vi "Nonlinear Lev-Mar Fit.vi"(5 "derivative":T2(ring), 6 "Standard Deviation":dbl[](array[numeric]) format="%0.2f", 7 "max iteration":i32=200, 8 "Initial Guess Coefficients":dbl[](array[numeric]) format="%0.2f", 9 "Y":dbl[](array[numeric]) format="%0.2f", 10 "X":dbl[](array[numeric]) format="%0.2f") -> (0 "error":i32, 1 "mse":dbl format="%0.4e", 2 "Best Fit":dbl[](array[numeric]) format="%0.2f", 3 "Best Fit Coefficients":dbl[](array[numeric]) format="%0.2f", 4 "Covariance":T1)   [LabVIEW 2014, in "NI_AALPro.lvlib"]
doc: "LabVIEW no longer supports this VI. Use the Nonlinear Curve Fit VI instead.\n\nUses the Levenberg-Marquardt algorithm to determine the least squares set of coefficients that best fit the set of input data points (X,Y) as expressed by a nonlinear function y=f(x,a), where a is the set of coefficients.\n\nUnlike the Levenberg Marquardt VI, you cannot wire formula strings representing models directly to this VI. You have to specify the nonlinear functions within a subVI of this VI. If you can express the models as formula strings, use the Levenberg Marquardt VI. If the Levenberg Marquardt VI takes too long to run because you have a large number of points, or if you cannot express your models as formula strings, use the Nonlinear Lev-Mar Fit VI instead.\n\nThis VI assumes that you have prior knowledge of the nonlinear relationship between the x and y coordinates. That is, f = f(X, A), where the set of coefficients, A, is determined by the Levenberg-Marquardt algorithm.\n\nIf your values of x are too large, consider normalizing them before applying them to this VI.\n\nYou must specify the nonlinear function f = f(X, A) in the Formula Node on the block diagram of the Target Fnc & Deriv NonLin VI, which is a subVI of the Nonlinear Lev-Mar Fit VI. To access the Target Fnc & Deriv NonLin VI, select <b>View>>Browse Relationships>>This VI's SubVIs>>Target Fnc & Deriv NonLin.vi</b>.\n\nThis VI provides the following two methods to calculate the Jacobian (partial derivatives with respect to the coefficients) needed in the algorithm:\n<b>numerical calculation</b> uses a numerical approximation to compute the Jacobian.\n<b>formula calculation</b> uses a formula to compute the Jacobian. You need to specify the Jacobian function df/dA in the Formula Node on the block diagram of the Target Fnc & Deriv NonLin VI, as well as the nonlinear function f = f(X, A) This is a more efficient computation than the numerical calculation, because it does not require a numerical approximation to the Jacobian."
uses:
  NI_AALPro.lvlib
  RealMatrix.ctl
  Real Inverse Matrix.vi
  NI_AALBase.lvlib
  NI_Matrix.lvlib
panel:
  # "Nonlinear  Lev-Mar  Fit"
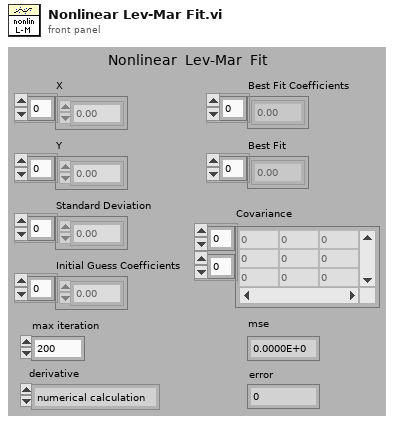
[diagram p1: front panel]
types:
  T1 = typedef "NI_Matrix.lvlib/RealMatrix.ctl" = dbl[][]
  T2 = enum32{"numerical calculation", "formula calculation"}
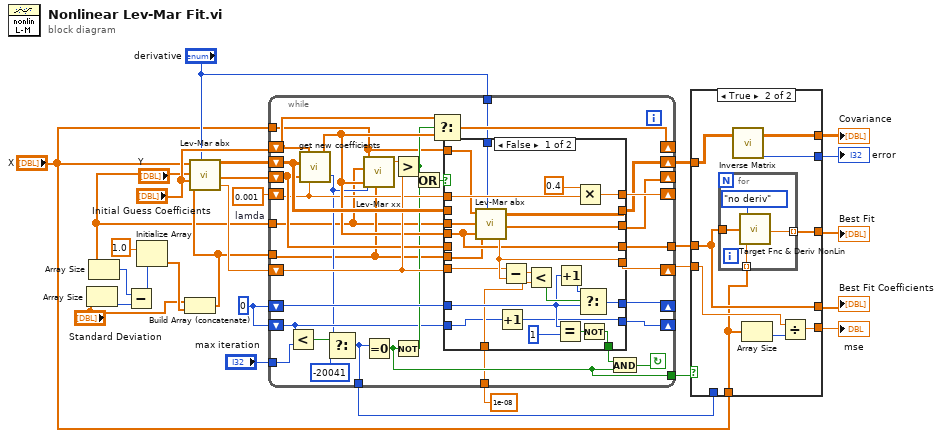
[diagram p0: block diagram]
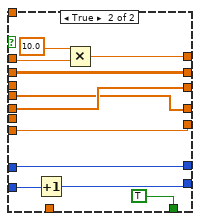
[diagram p2: hidden frame]
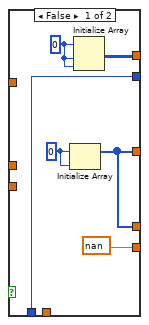
[diagram p3: hidden frame]
diagram:
  w18 = 0
  w27 = 0.001  # lamda
  n1 = Array Size(array="Standard Deviation") -> (size(s)=w8:i32)
  n2 = Array Size(array="Y") -> (size(s)=w9:i32)
  n3 = Subtract(x=w9, y=w8) -> (x-y=w7:i32)
  n4 = Initialize Array(1.0, w7) -> (w6:dbl[])
  n5 = Build Array (concatenate)("Standard Deviation", w6) -> (w4:dbl[])
  n6 = call "Lev-Mar abx.vi"("X"="X", "Y"="Y", "Coefficients"="Initial Guess Coefficients", "Standard Deviation"=w4, "derivative"="derivative") -> ("Alpha"=w28:dbl[][], "Beta"=w26:dbl[], "chiSqr"=w25:dbl)
  n7 = while {
    tunnel: "X" -> [w30]
    tunnel: "Y" -> [w32]
    tunnel: [w33] -> w11
    tunnel: "max iteration" -> [w35]
    tunnel: w4 -> [w34]
    shift-left: w18 -> [w39]
    shift-right: [w40] -> _
    tunnel: 1e-08 -> [w44]
    tunnel: [w45] -> w20
    tunnel: [w48] -> w23
    shift-left: w18 -> [w53]
    shift-right: [w52] -> _
    shift-left: w25 -> [w54]
    shift-right: [w55] -> w24
    shift-left: w26 -> [w51]
    shift-right: [w56] -> _
    shift-left: w28 -> [w57]
    shift-right: [w58] -> w10
    shift-left: "Initial Guess Coefficients" -> [w31]
    shift-right: [w59] -> _
    shift-left: w27 -> [w49]
    shift-right: [w60] -> _
    tunnel: "derivative" -> [w29]
    stop <- w47 continue-if-true
    n8 = Less?(x=w39, y=w35) -> (x < y?=w38:bool)
    n9 = call "get new coefficients.vi"("lamda"=w49, "Beta"=w51, "Alpha"=w57, "Coefficients"=w31) -> ("error"=w36:i32, "New Coefficients"=w50:dbl[])
    n10 = Select(t=w36, s=w38, f=-20041) -> (s? t:f=w33:i32)
    n11 = call "Lev-Mar xx.vi"("X"=w30, "Y"=w32, "Coefficients"=w50, "error"=w36, "Standard Deviation"=w34) -> ("chiSqr"=w61:dbl)
    n12 = Equal To 0?(x=w33) -> (x = 0?=w45:bool)
    n13 = Greater?(x=w61, y=w54) -> (0:w42:bool)
    n14 = Not(x=w45) -> (.not. x?=w41:bool)
    n15 = Or(x=w42, y=w41) -> (x .or. y?=w43:bool)
    n16 = Select(t=w31, s=w42, f=w50) -> (s? t:f=w59:dbl[])
    n17 = case shown="False" w43 {
      tunnel: w49 -> [w83 w94]
      tunnel: [w82 w93] -> w60
      tunnel: [w81 w92] -> w58
      tunnel: w57 -> [_ w92]
      tunnel: [w80 w88] -> w56
      tunnel: [w79 w91] -> w55
      tunnel: w54 -> [w78 w91]
      tunnel: w53 -> [w73 w90]
      tunnel: [w74 w90] -> w52
      tunnel: [w70 TRUE] -> w46
      tunnel: w50 -> [w67 w87]
      tunnel: w51 -> [_ w88]
      tunnel: [w67 w87] -> w48
      tunnel: w44 -> [w69 _]
      tunnel: [w65 w86] -> w40
      tunnel: w39 -> [w68 w85]
      tunnel: w34 -> [w66 _]
      tunnel: w30 -> [w64 _]
      tunnel: w32 -> [w63 _]
      tunnel: w29 -> [w62 _]
      frame False {
        n18 = call "Lev-Mar abx.vi"("X"=w64, "Y"=w63, "Coefficients"=w67, "Standard Deviation"=w66, "derivative"=w62) -> ("Alpha"=w81:dbl[][], "Beta"=w80:dbl[], "chiSqr"=w79:dbl)
        n19 = Increment(x=w68) -> (x+1=w65:i32)
        n20 = Subtract(x=w78, y=w79) -> (x-y=w77:dbl)
        n21 = Less?(x=w77, y=w69) -> (x < y?=w76:bool)
        n22 = Equal?(x=w73, y=1) -> (x = y?=w71:bool)
        n23 = Increment(x=w73) -> (x+1=w75:i32)
        n24 = Multiply(x=0.4, y=w83) -> (x*y=w82:dbl)
        n25 = Select(t=w75, s=w76, f=w73) -> (s? t:f=w74:i32)
        n26 = Not(x=w71) -> (.not. x?=w70:bool)
      }
      frame True {
        n27 = Increment(x=w85) -> (x+1=w86:i32)
        n28 = Multiply(x=10.0, y=w94) -> (x*y=w93:dbl)
      }
    }
    n29 = And(x=w46, y=w45) -> (x .and. y?=w47:bool)
  }
  n30 = case shown="True" w20 {
    tunnel: w23 -> [_ w107]
    tunnel: [w99 w107] -> w22
    tunnel: [nan w110] -> w21
    tunnel: [w99 w108] -> w14
    tunnel: w24 -> [_ w106]
    tunnel: [w97 w105] -> w13
    tunnel: [w96 w104] -> w12
    tunnel: w11 -> [w96 _]
    tunnel: w10 -> [_ w103]
    tunnel: "X" -> [_ w102]
    frame False {
      w98 = 0
      w101 = 0
      n31 = Initialize Array(w101, w101) -> (w99:i32[])
      n32 = Initialize Array(w98, w98, w98) -> (w97:i32[][])
    }
    frame True {
      n33 = for {
        tunnel: w107 -> [w113]
        tunnel: [w112] -> w108 mode=indexing
        tunnel: w102 -> [w114] mode=indexing
        n34 = call "Target Fnc & Deriv NonLin.vi"("X"=w114, "Coefficients"=w113, "Flag"=enum16{"no deriv", "deriv"}."no deriv") -> ("Y"=w112:dbl)  [unwired: 1 out]
      }
      n35 = call-poly "Inverse Matrix.vi"("Input Matrix"=w103) -> ("error"=w104:i32, "Inverse Matrix"=w105:T1)  [unwired: 1 in]
      n36 = Array Size(array=w102) -> (size(s)=w109:i32)
      n37 = Divide(x=w106, y=w109) -> (x/y=w110:dbl)
    }
  }
  "mse" <- w21
  "Best Fit Coefficients" <- w22
  "Best Fit" <- w14
  "error" <- w12
  "Covariance" <- w13
